vi "LCP Get Pump Name.vi"(8 "error in (no error)":errorcluster caption="Fehler (Eingang, kein Fehler)", 11 "Pump Handle":i64) -> (0 "error out":errorcluster caption="Fehler (Ausgang)", 3 "Pump Name":string)   [LabVIEW 2023, in "labbCAN_Pump_API.lvlib"]
doc: "LCP_Func long LCP_CALL LCP_GetPumpName(dev_hdl hPump,\n char *pNameStringBuf,\n int StringBufSize);"
uses:
  labbCAN_Pump_API.lvlib
  labbCAN_Pump_API.dll
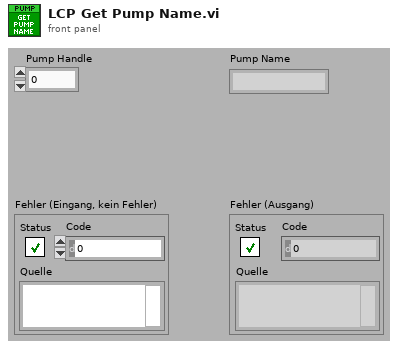
[diagram p1: front panel]
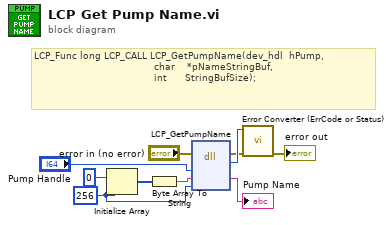
[diagram p0: block diagram]
diagram:
  w1 = 256 ("Dimension")
  # "LCP_Func long LCP_CALL LCP_GetPumpName(dev_hdl  hPump,\n                                        char    *pNameStringBuf,\n                                        int      StringBufSize);"
  n1 = Initialize Array(u8 0 ("Element"), w1) -> (w9:u8[])
  n2 = Byte Array To String(unsigned byte array=w9) -> (string=w8:string)
  n3 = dll-call lib="C:/GIT/DensityGradientProject/CETONI_SDK/labbCAN_Pump_API.*" fn="LCP_GetPumpName"(error in="error in (no error)", "hPump"="Pump Handle", "pNameStringBuf"=w8, "StringBufSize"=w1) -> (error out=w3:errorcluster, "Rückgabetyp"=w4:i32, "pNameStringBuf"=→"Pump Name":string)  [unwired: 4 in, 1 out]
  n4 = call "Error Converter (ErrCode or Status).vi"("error in (no error)"=w3, "error code"=w4) -> ("error out"=→"error out":errorcluster)  [unwired: 9 in]
